vi "test_Write FXP Register Value_Lower Than Minimum.vi"(8 "error in (no error)":errorcluster, 11 "TestCase in":refnum<class "FPGA Register IO Tests.lvclass">) -> (0 "error out":errorcluster, 3 "TestCase out":refnum<class "FPGA Register IO Tests.lvclass">)   [LabVIEW 2021, in "FPGA Register IO Tests.lvclass"]
uses:
  FPGA Register IO Tests.lvclass
  APIs/FPGA Register IO/TypeDefs/FXP Configuration.ctl
  <vilib>/fxp/LVFixedPointRepBitsTypeDef.ctl
  <vilib>/fxp/LVFixedPointRepRangeTypeDef.ctl
  FPGA Register IO Tests.lvclass/FPGA Register IO Tests.ctl
  APIs/FPGA Register IO/Write Methods/Write Data Register/Instances/Write FXP.vi
  APIs/FPGA Register IO/Read Methods/Read Data Register/Instances/Read FXP.vi
  APIs/FPGA Register IO/Write Methods/Write Data Register/Instances/Write U8.vi
  APIs/FPGA Register IO/Write Methods/Write Data Register/Instances/Write U16.vi
  APIs/FPGA Register IO/Write Methods/Write Data Register/Instances/Write U32.vi
  APIs/FPGA Register IO/Write Methods/Write Data Register/Instances/Write U64.vi
  APIs/FPGA Register IO/SubVIs/DBL to FXP Raw.vi
  APIs/FPGA Register IO/SubVIs/FXP Raw to DBL.vi
  APIs/FPGA Register IO/Read Methods/Read Data Register/Instances/Read U8.vi
  APIs/FPGA Register IO/Read Methods/Read Data Register/Instances/Read U16.vi
  APIs/FPGA Register IO/Read Methods/Read Data Register/Instances/Read U32.vi
  APIs/FPGA Register IO/Read Methods/Read Data Register/Instances/Read U64.vi
  APIs/FPGA Register IO/Utilities/Find Register Offset.vi
  APIs/FPGA Register IO/SubVIs/Check Register Data Store.vi
  APIs/FPGA Register IO/Error Handling/Error 6001.vi
  APIs/FPGA Register IO/Error Handling/Error 6000.vi
  APIs/FPGA Register IO/Error Handling/Error 6002.vi
  APIs/FPGA Register IO/Error Handling/Error 6006.vi
  APIs/FPGA Register IO/Error Handling/Error 6003.vi
  <vilib>/FPGAPlugInAG/Dynamic/niLvFpga_Close_Dynamic.vi
  <vilib>/rvi/interface/nirviCloseFPGA/nirviCloseFPGA.xnode
  <vilib>/addons/_JKI Toolkits/VI Tester/TestCase.llb/TestCase.lvclass
  APIs/FPGA Register IO/FPGA Register IO.lvlib
  <vilib>/Utility/Data Type/NI_Data Type.lvlib
  C:/Program Files/National Instruments/LabVIEW 2021/vi.lib/addons/_JKI Toolkits/VI Tester/TestCase.llb/TestCase.lvclass
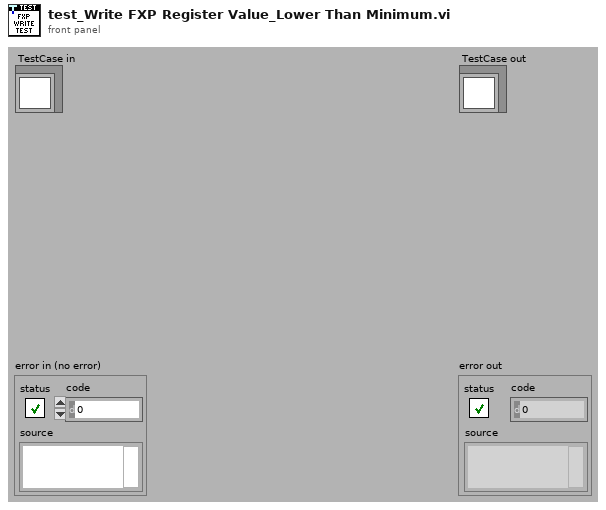
[diagram p1: front panel]
types:
  T1 = typedef "FPGA Register IO.lvlib/FXP Configuration.ctl" = cluster{"FXP Representation":T2, "FXP Range":T3}
  T2 = typedef "LVFixedPointRepBitsTypeDef.ctl" = cluster{"Signed":bool, "Word Length":u32, "Integer Word Length":i32}
  T3 = typedef "LVFixedPointRepRangeTypeDef.ctl" = cluster{"Range Min":dbl, "Range Max":dbl, "Delta":dbl}
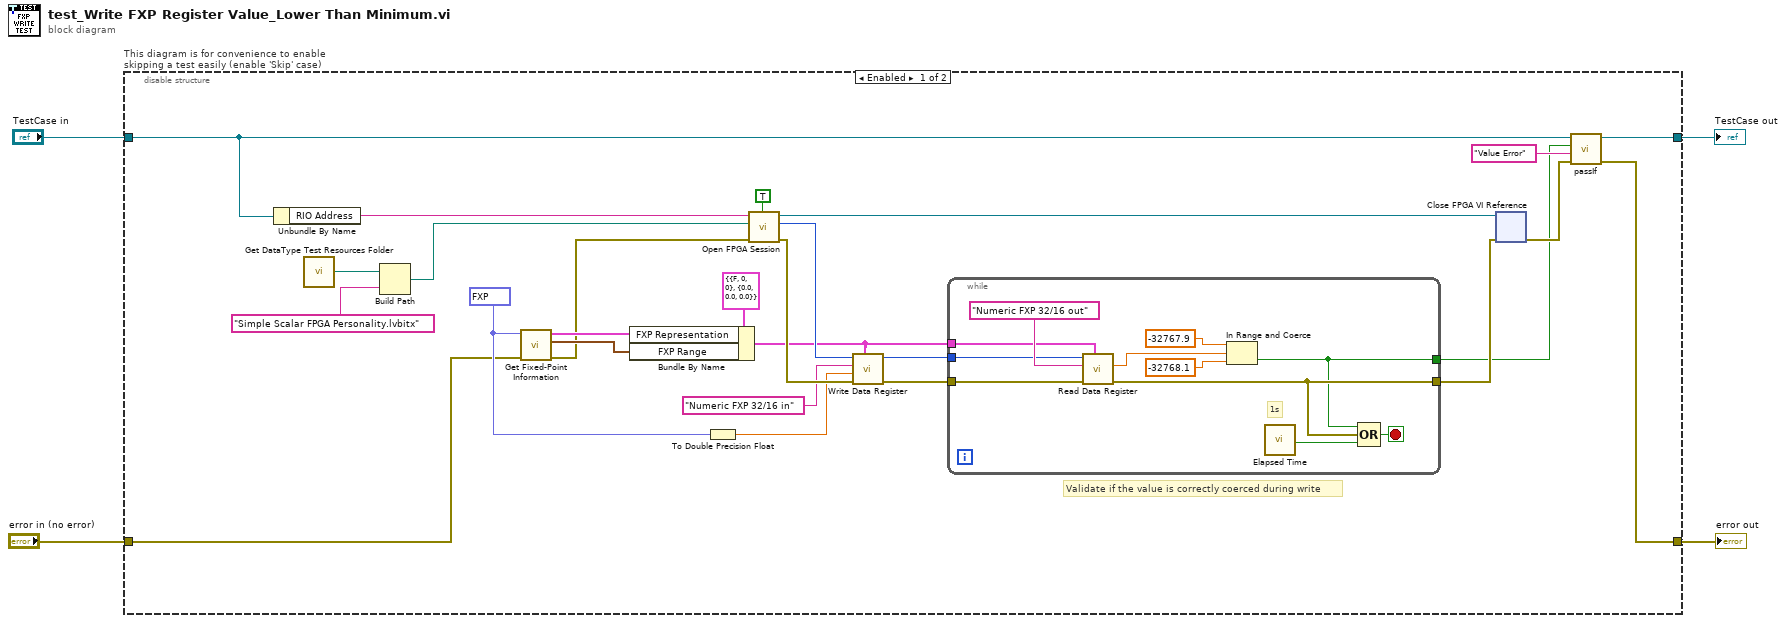
[diagram p0: block diagram]
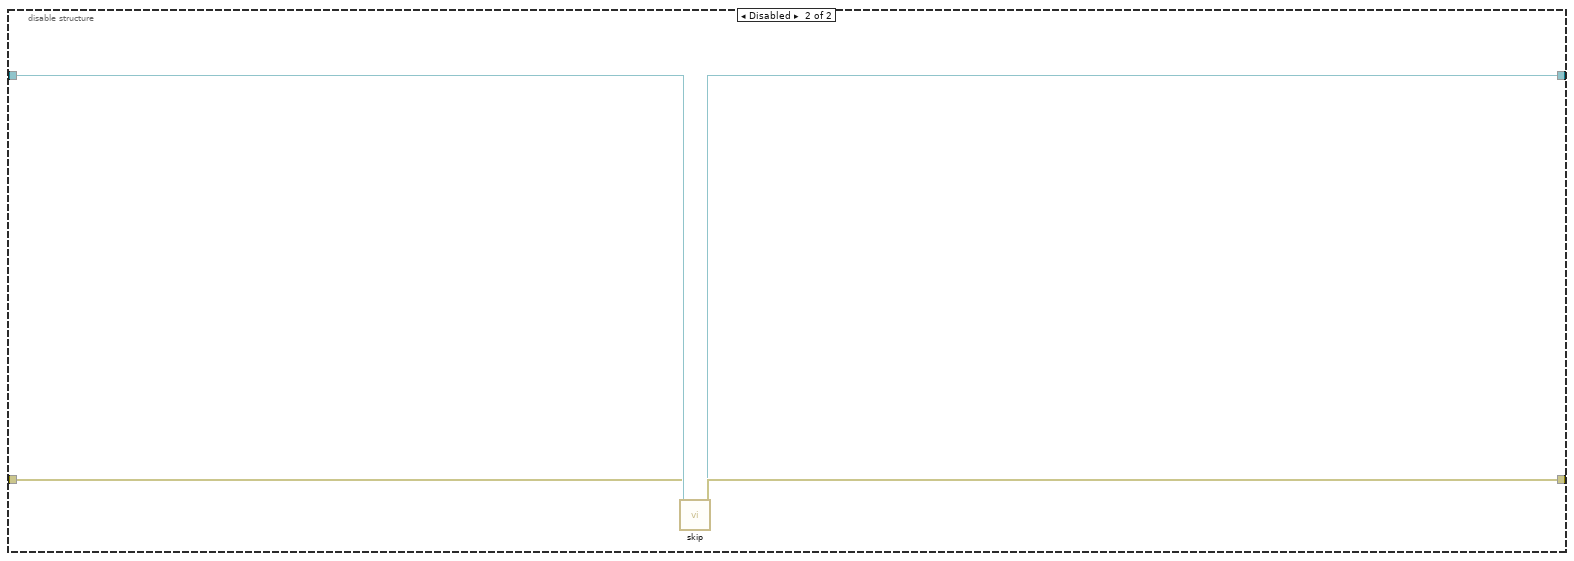
[diagram p2: hidden frame]
diagram:
  n1 = disable-structure "This diagram is for convenience to enable skipping a test easily (enable 'Skip' case)" shown="Enabled" {
    disable-tunnel: "TestCase in" -> [w26 w45]
    disable-tunnel: [w22 w43] -> w1
    disable-tunnel: [w21 w44] -> w3
    disable-tunnel: "error in (no error)" -> [w7 w42]
    frame Enabled {
      w9 = fxp<+/-,32,16> -32768.0 ("value in")
      # "Validate if the value is correctly coerced during write"
      n2 = Unbundle By Name(w26) -> ("RIO Address"=w20:string)
      n3 = call "Get DataType Test Resources Folder.vi"() -> ("path"=w24:path)
      n4 = Build Path(base path=w24, name or relative path="Simple Scalar FPGA Personality.lvbitx") -> (appended path=w27:path)
      n5 = call <vilib>:"Get Fixed-Point Information.vi"("error in (no error)"=w7, "variant"=w9) -> ("error out"=w6:errorcluster, "FXP range"=w11:T3, "FXP representation"=w12:T2)  [unwired: 6 in, 1 out]
      n6 = Bundle By Name(cluster=T1 {"FXP Representation"={"Signed"=FALSE, "Word Length"=0, "Integer Word Length"=0}, "FXP Range"={"Range Min"=0.0, "Range Max"=0.0, "Delta"=0.0}} ("FXP Configuration"), "FXP Representation"=w12, "FXP Range"=w11) -> (w5:T1)
      n7 = To Double Precision Float(number=w9) -> (double precision float=w8:dbl)
      n8 = call "Open FPGA Session.vi"("run when loaded (T)"=TRUE ("Run When Loaded (T)"), "error in"=w6, "bitfile path"=w27, "device address"=w20) -> ("error out"=w19:errorcluster, "session out"=w17:u32, "bitfile reference out"=w29:refnum<k20>)  [unwired: 5 in]
      n9 = call-poly "Write Data Register.vi"("FXP Configuration"=w5, "error in"=w19, "DBL Value"=w8, "register name"="Numeric FXP 32/16 in", "session in"=w17) -> ("error out"=w15:errorcluster, "session out"=w16:u32)  [unwired: 5 in]
      n10 = while {
        tunnel: [w37] -> w14
        tunnel: w15 -> [w40]
        tunnel: w16 -> [w39]
        tunnel: w5 -> [w35]
        tunnel: [w34] -> w13
        stop <- w38 stop-if-true
        # "1s"
        n11 = call-poly "Read Data Register.vi"("FXP Configuration"=w35, "error in"=w40, "register name"="Numeric FXP 32/16 out" ("registerName"), "session in"=w39) -> ("error out"=w37:errorcluster, "DBL Value"=w33:dbl)  [unwired: 5 in, 1 out]
        n12 = In Range and Coerce(upper limit=-32767.9 ("y"), x=w33, lower limit=-32768.1 ("y")) -> (In Range?=w34:bool)  [unwired: 1 out]
        n13 = call "Elapsed Time"() -> ("Time has Elapsed"=w36:bool)  [unwired: 12 in, 7 out]
        n14 = Compound Arithmetic op=OR(w34, w37, w36) -> (w38:bool)
      }
      n15 = xnode "Close FPGA VI Reference"("FPGA VI Reference In"=w29, "error in"=w14) -> ("error out"=w25:errorcluster)
      n16 = call-dynamic "passIf.vi"("error in (no error)"=w25, "message (\"\")"="Value Error" ("message (\"\")"), "pass"=w13, "TestCase in"=w26) -> ("error out"=w21:errorcluster, "TestCase out"=w22:refnum<class "FPGA Register IO Tests.lvclass">)  [unwired: 6 in]
    }
    frame Disabled {
      # "skip test result while test is under development"
      n17 = call <vilib>:"skip.vi"("error in (no error)"=w42, "TestCase in"=w45) -> ("error out"=w44:errorcluster, "TestCase out"=w43:refnum<class "FPGA Register IO Tests.lvclass">)  [unwired: 8 in]
    }
  }
  "error out" <- w3
  "TestCase out" <- w1
